vi "LCD Print.vi"(8 "Error In":errorcluster, 9 "Base (String)":T4, 10 "Data":string, 11 "ChipKit Resource":T1={"COM Port"="", "Board Type"=enum."ChipKit Uno32", "Connection Type"=enum."USB / Serial", "Baud Rate (115200)"=0, "Bytes Per Packet (15)"=15, "DI Port Num Pins"=0, "DO Port Num Pins"=0}) -> (0 "Error Out":errorcluster, 3 "ChipKit Resource":T1={"COM Port"="", "Board Type"=enum."ChipKit Uno32", "Connection Type"=enum."USB / Serial", "Baud Rate (115200)"=0, "Bytes Per Packet (15)"=15, "DI Port Num Pins"=0, "DO Port Num Pins"=0})   [LabVIEW 2011, in "LabVIEW Interface for ChipKit.lvlib"]
doc: "Prints data of the specified type to the LCD screen."
uses:
  LabVIEW Interface for ChipKit.lvlib
  Private/Type Defs/Base.ctl
  Private/Type Defs/Chipkit Resource.ctl
  Private/Type Defs/Board Type.ctl
  Private/Type Defs/Connection Type.ctl
  Private/Type Defs/Command.ctl
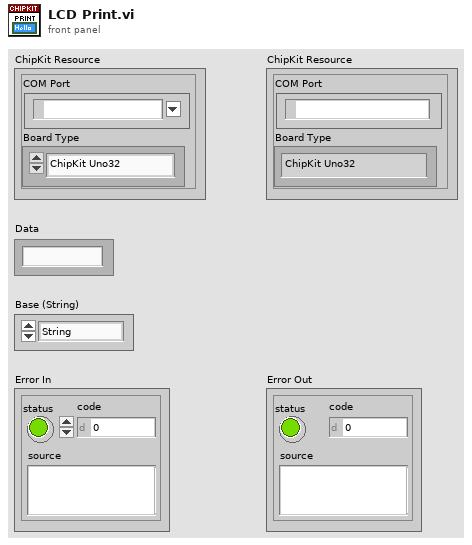
[diagram p1: front panel]
types:
  T1 = typedef "LabVIEW Interface for ChipKit.lvlib/Chipkit Resource.ctl" = cluster{"COM Port":refnum<visa-resource-name>, "Board Type":T2, "Connection Type":T3, "Baud Rate (115200)":u32, "Bytes Per Packet (15)":u32, "DI Port Num Pins":i32, "DO Port Num Pins":i32}
  T2 = typedef "LabVIEW Interface for ChipKit.lvlib/Board Type.ctl" = enum16{"ChipKit uC32", "ChipKit Uno32", "ChipKit Max32"}
  T3 = typedef "LabVIEW Interface for ChipKit.lvlib/Connection Type.ctl" = enum8{"USB / Serial", "XBEE", "BlueSmirf (Bluetooth)"}
  T4 = typedef "LabVIEW Interface for ChipKit.lvlib/Base.ctl" = enum16{"String", "Binary", "Decimal", "Octal", "Hexadecimal"}
  T5 = typedef "LabVIEW Interface for ChipKit.lvlib/Command.ctl" = enum8{"setArduinoMode", "flushSerial", "setPinMode", "digitalWritePin", "digitalWritePort", "tone", "digitalReadPin", "digitalReadPort", "analogReadPin", "analogReadPort", "pwmWritePin", "pwmWritePort", "sevenSegment_Configure", "sevenSegment_Write", "I2C Init", "I2C Write", "I2C Read", "SPI Init", "SPI Set Bit Order", "SPI Set Clock Divider", "SPI Set Data Mode", "SPI Send / Receive", "SPI Close", "Servo Set Num Servos", "Servo Config Servo", "Servo Write Angle", "Servo Read Angle", "Servo Write Pulse Width", "Servo Read Pulse Width", "Servo Detach", "LCD Init", "LCD Set Size", "LCD Set Cursor Mode", "LCD Clear", "LCD Set Cursor Position", "LCD Print", "LCD Display Power", "LCD Scroll Display", "LCD Autoscroll", "LCD Print Direction", "LCD Create Custom Char", "LCD Print Custom Char", "contAcqOn", "contAcqOff", "getFirmwareVersion", "FiniteSampleStart", "NA", "NA2", "Conifg Stepper", "Stepper Write", "Stepper Detach", "Stepper Steps To Go", "Config DO Port", "Config DI Port"}
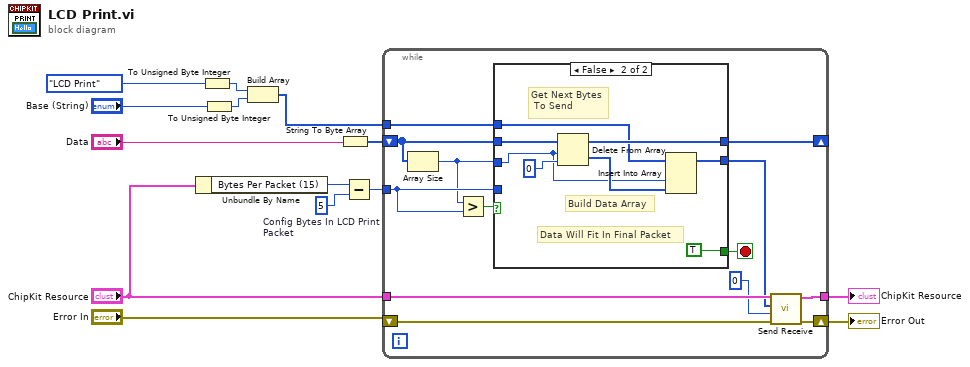
[diagram p0: block diagram]
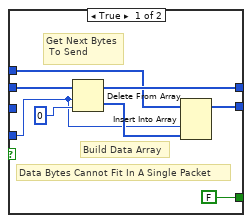
[diagram p2: hidden frame]
diagram:
  w6 = u8 5  # Config Bytes In LCD Print Packet
  n1 = Unbundle By Name("ChipKit Resource") -> ("Bytes Per Packet (15)"=w2:u32)
  n2 = To Unsigned Byte Integer(number=Command."LCD Print" ("Command")) -> (unsigned 8bit integer=w10:u8)
  n3 = To Unsigned Byte Integer(number="Base (String)") -> (unsigned 8bit integer=w3:u8)
  n4 = Build Array(w10, w3) -> (w1:u8[])
  n5 = String To Byte Array(string="Data") -> (unsigned byte array=w5:u8[])
  n6 = Subtract(x=w2, y=w6) -> (x-y=w4:u32)
  n7 = while {
    tunnel: [w26] -> w13
    tunnel: "ChipKit Resource" -> [w24]
    shift-right: [w27] -> w14
    shift-left: "Error In" -> [w25]
    shift-right: [w22] -> _
    shift-left: w5 -> [w18]
    tunnel: w4 -> [w17]
    tunnel: w1 -> [w21]
    stop <- w15 stop-if-true
    n8 = Array Size(array=w18) -> (size(s)=w16:i32)
    n9 = Greater?(x=w16, y=w17) -> (0:w19:bool)
    n10 = case shown="False" w19 {
      tunnel: w18 -> [w35 w43]
      tunnel: w17 -> [w28 _]
      tunnel: [w33 w41] -> w22
      tunnel: w21 -> [w32 w40]
      tunnel: [w31 w39] -> w20
      tunnel: w16 -> [_ w36]
      tunnel: [FALSE TRUE] -> w15
      frame True {
        # "Data Bytes Cannot Fit In A Single Packet"
        # "Build Data Array"
        # "Get Next Bytes\n To Send"
        n11 = Delete From Array(array=w35, length=w28, index=0) -> (deleted portion=w29:u8[], array with subset deleted=w33:u8[])
        n12 = Insert Into Array(array=w32, new element #1=w28, new element #2=w29) -> (w31:u8[])  [unwired: 1 in]
      }
      frame False {
        # "Data Will Fit In Final Packet"
        # "Build Data Array"
        # "Get Next Bytes\n To Send"
        n13 = Delete From Array(array=w43, length=w36, index=0) -> (deleted portion=w37:u8[], array with subset deleted=w41:u8[])
        n14 = Insert Into Array(array=w40, new element #1=w36, new element #2=w37) -> (w39:u8[])  [unwired: 1 in]
      }
    }
    n15 = call "Send Receive.vi"("Error In"=w25, "Bytes To Read (0)"=u8 0, "Data"=w20, "ChipKit Resource"=w24) -> ("Error Out"=w27:errorcluster, "ChipKit Resource"=w26:T1)  [unwired: 5 in, 1 out]
  }
  "Error Out" <- w14
  "ChipKit Resource" <- w13
